vi "Aquisition_Reactor_Coolant_Loop_Temperature_SG_Outlet.vi"(0 "SI101_AverageReactorCoolantTemperature.lvclass":refnum<class "SI101.lvclass">, 1 "3 JEC10 CT001A XQ01":dbl, 2 "3 JEC20 CT001A XQ01":dbl, 3 "3 JEC30 CT001A XQ01":dbl, 4 "3 JEC40 CT001A XQ01":dbl, 5 "error in (no error)":errorcluster, 7 "In1":dbl=4.0, 9 "In2":dbl=20.0) -> (14 "SI101_AverageReactorCoolantTemperature.lvclass out":refnum<class "SI101.lvclass">, 15 "JEC10CT001A":dbl, 16 "JEC20CT001A":dbl, 17 "JEC30CT001A":dbl, 18 "JEC40CT001A":dbl, 19 "error IO":errorcluster)   [LabVIEW 2022 SP3, in "SI101.lvclass"]
uses:
  SI101.lvclass
  SI101.lvclass/SI101.ctl
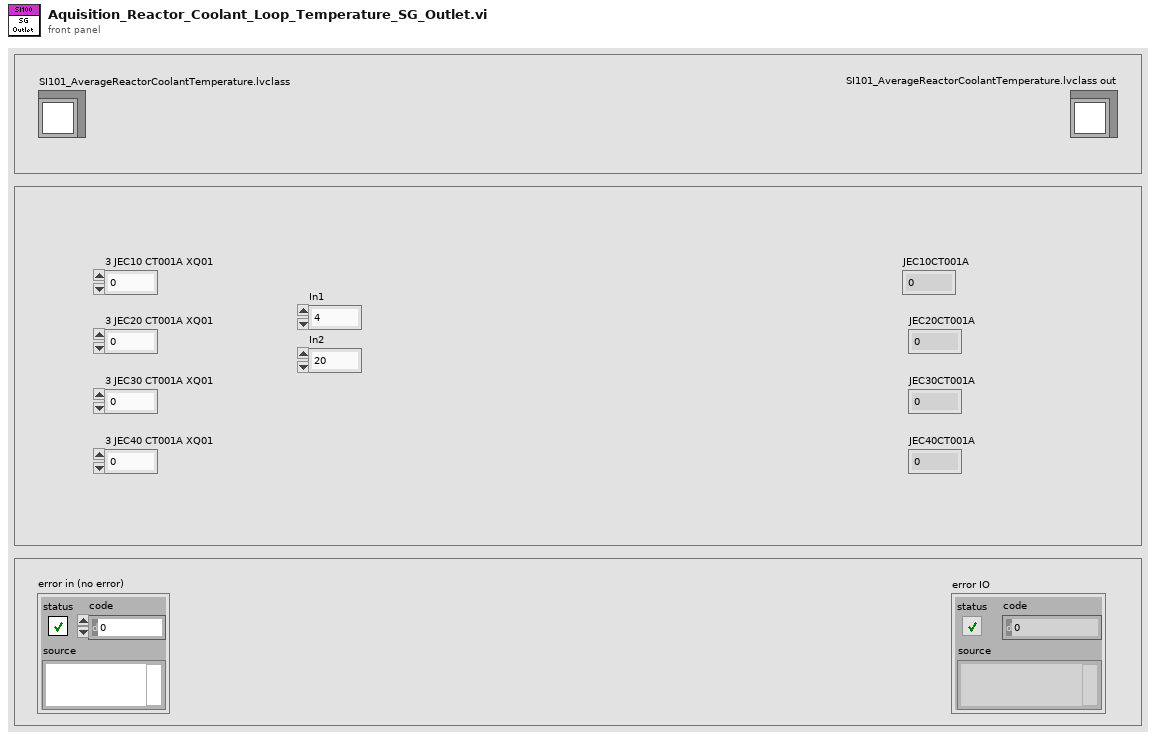
[diagram p1: front panel]
types:
  T1 = cluster{"LL":dbl, "OutLimMin":dbl, "OutLimMax":dbl, "UL":dbl, "In1":dbl, "In2":dbl, "Out1":dbl, "Out2":dbl, "Limitation":bool}
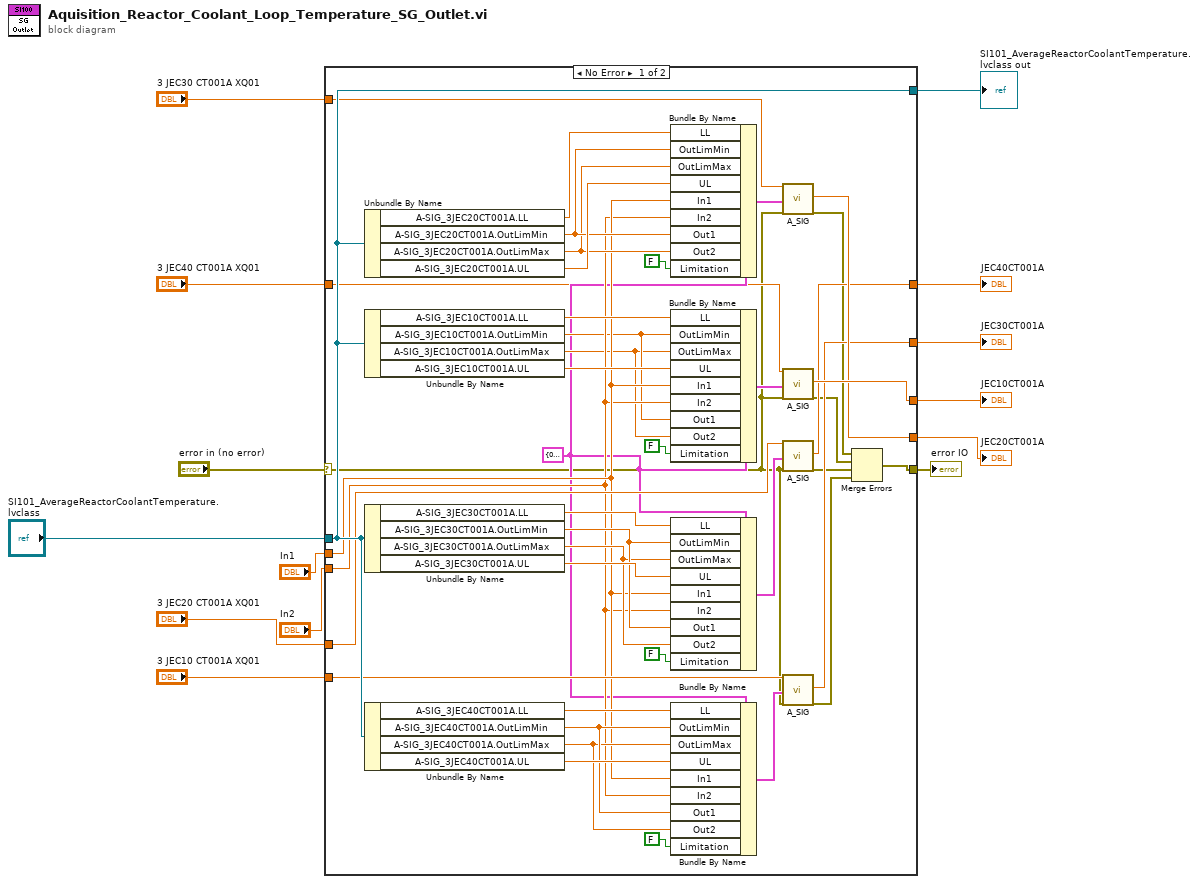
[diagram p0: block diagram]
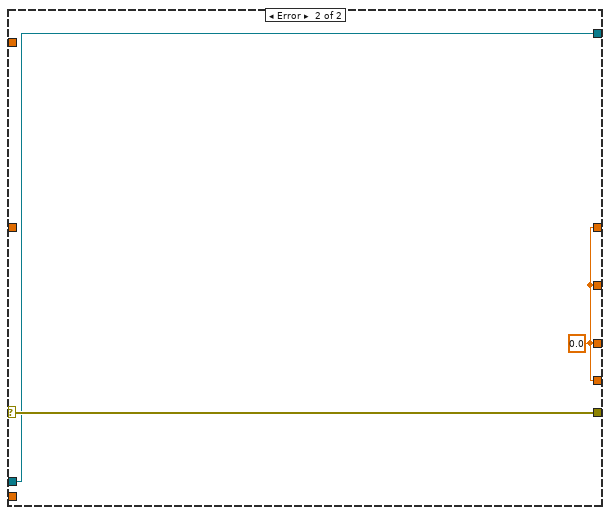
[diagram p2: hidden frame]
diagram:
  n1 = case shown="No Error" "error in (no error)" {
    selector: "error in (no error)" -> [w20 w59]
    tunnel: [w15 w59] -> w13
    tunnel: "3 JEC10 CT001A XQ01" -> [w46 _]
    tunnel: "3 JEC20 CT001A XQ01" -> [w40 _]
    tunnel: "3 JEC30 CT001A XQ01" -> [w31 _]
    tunnel: "3 JEC40 CT001A XQ01" -> [w21 _]
    tunnel: [w56 w58] -> w8
    tunnel: "SI101_AverageReactorCoolantTemperature.lvclass" -> [w56 w58]
    tunnel: [w55 w57] -> w6
    tunnel: [w54 w57] -> w5
    tunnel: [w53 w57] -> w4
    tunnel: [w52 w57] -> w3
    tunnel: "In1" -> [w28 _]
    tunnel: "In2" -> [w27 _]
    frame No Error {
      w23 = T1 {"LL"=0.0, "OutLimMin"=0.0, "OutLimMax"=0.0, "UL"=0.0, "In1"=0.0, "In2"=0.0, "Out1"=0.0, "Out2"=0.0, "Limitation"=FALSE} ("Cluster")
      n2 = Unbundle By Name(w56) -> ("A-SIG_3JEC20CT001A.LL"=w38:dbl, "A-SIG_3JEC20CT001A.OutLimMin"=w36:dbl, "A-SIG_3JEC20CT001A.OutLimMax"=w35:dbl, "A-SIG_3JEC20CT001A.UL"=w37:dbl)
      n3 = Unbundle By Name(w56) -> ("A-SIG_3JEC10CT001A.LL"=w30:dbl, "A-SIG_3JEC10CT001A.OutLimMin"=w26:dbl, "A-SIG_3JEC10CT001A.OutLimMax"=w25:dbl, "A-SIG_3JEC10CT001A.UL"=w29:dbl)
      n4 = Unbundle By Name(w56) -> ("A-SIG_3JEC30CT001A.LL"=w45:dbl, "A-SIG_3JEC30CT001A.OutLimMin"=w43:dbl, "A-SIG_3JEC30CT001A.OutLimMax"=w42:dbl, "A-SIG_3JEC30CT001A.UL"=w44:dbl)
      n5 = Unbundle By Name(w56) -> ("A-SIG_3JEC40CT001A.LL"=w51:dbl, "A-SIG_3JEC40CT001A.OutLimMin"=w49:dbl, "A-SIG_3JEC40CT001A.OutLimMax"=w48:dbl, "A-SIG_3JEC40CT001A.UL"=w50:dbl)
      n6 = Bundle By Name(cluster=w23, "LL"=w38, "OutLimMin"=w36, "OutLimMax"=w35, "UL"=w37, "In1"=w28, "In2"=w27, "Out1"=w36, "Out2"=w35, "Limitation"=FALSE) -> (w32:T1)
      n7 = Bundle By Name(cluster=w23, "LL"=w30, "OutLimMin"=w26, "OutLimMax"=w25, "UL"=w29, "In1"=w28, "In2"=w27, "Out1"=w26, "Out2"=w25, "Limitation"=FALSE) -> (w22:T1)
      n8 = Bundle By Name(cluster=w23, "LL"=w45, "OutLimMin"=w43, "OutLimMax"=w42, "UL"=w44, "In1"=w28, "In2"=w27, "Out1"=w43, "Out2"=w42, "Limitation"=FALSE) -> (w39:T1)
      n9 = Bundle By Name(cluster=w23, "LL"=w51, "OutLimMin"=w49, "OutLimMax"=w48, "UL"=w50, "In1"=w28, "In2"=w27, "Out1"=w49, "Out2"=w48, "Limitation"=FALSE) -> (w47:T1)
      n10 = call "A_SIG.vi"("Input(AI1)"=w31, "Cluster"=w32, "error in (no error)"=w20) -> ("AO1"=w54:dbl, "error out"=w19:errorcluster)  [unwired: 13 in, 2 out]
      n11 = call "A_SIG.vi"("Input(AI1)"=w21, "Cluster"=w22, "error in (no error)"=w20) -> ("AO1"=w55:dbl, "error out"=w18:errorcluster)  [unwired: 13 in, 2 out]
      n12 = call "A_SIG.vi"("Input(AI1)"=w40, "Cluster"=w39, "error in (no error)"=w20) -> ("AO1"=w52:dbl, "error out"=w17:errorcluster)  [unwired: 13 in, 2 out]
      n13 = call "A_SIG.vi"("Input(AI1)"=w46, "Cluster"=w47, "error in (no error)"=w20) -> ("AO1"=w53:dbl, "error out"=w16:errorcluster)  [unwired: 13 in, 2 out]
      n14 = Merge Errors(w19, w18, w17, w16) -> (w15:errorcluster)
    }
    frame Error {
      w57 = 0.0 ("AO1")
    }
  }
  "error IO" <- w13
  "SI101_AverageReactorCoolantTemperature.lvclass out" <- w8
  "JEC10CT001A" <- w6
  "JEC20CT001A" <- w5
  "JEC30CT001A" <- w4
  "JEC40CT001A" <- w3
